vi "MeasureSave.vi"(7 "MinutesToWait":u32, 8 "Stop":bool, 9 "Number of Spectra":u16=1, 11 "Handle":u32) -> (1 "phase":dbl[](array[numeric]), 2 "mag":dbl[](array[numeric]), 3 "Freq":dbl[](array[numeric]), 4 "Current Incoming row":u16, 6 "SpecCount":u16)   [LabVIEW 2012]
uses:
  <vilib>/Utility/file.llb/Write To Spreadsheet File (DBL).vi
  Sciospec ISX3 Impedance Analyzer.lvlib
panel:
  out "ACK for Start CMD":u8[](array[numeric])
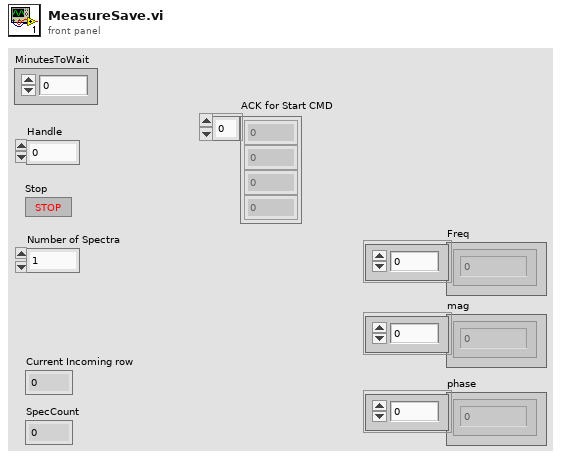
[diagram p1: front panel]
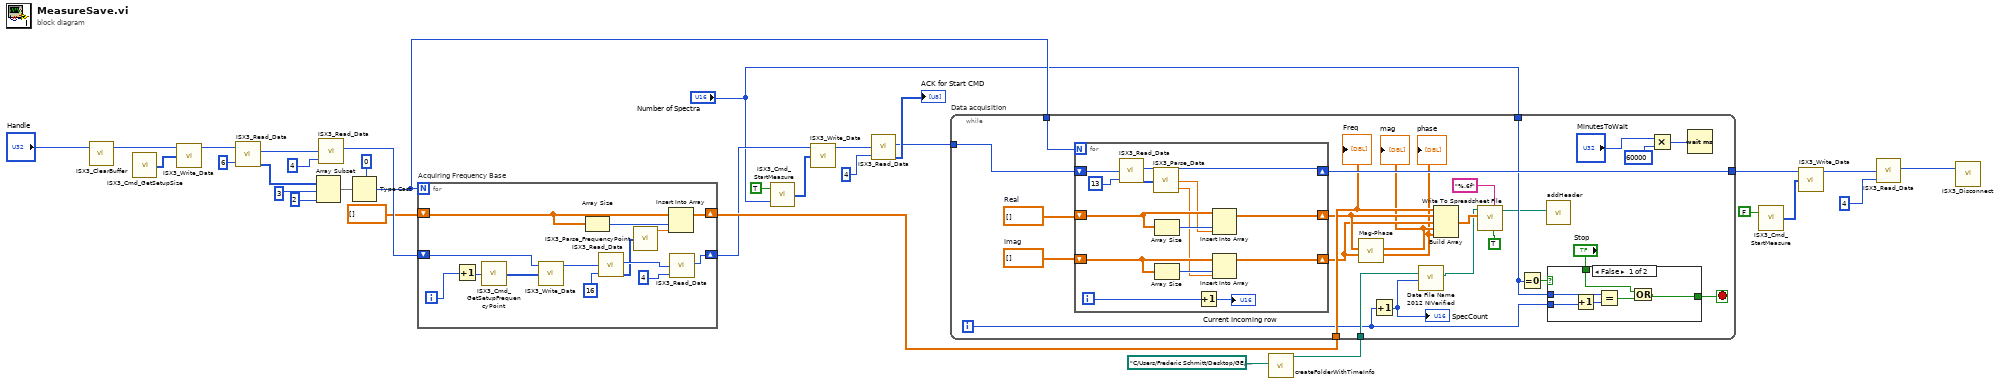
[diagram p0: block diagram]
diagram:
  n1 = call "ISX3_ClearBuffer.vi"("Handle"="Handle") -> ("Handle"=w4:u32)  [unwired: 1 in, 1 out]
  n2 = call "ISX3_Cmd_GetSetupSize.vi"() -> ("get Setup Size Cmd"=w15:u8[])  [unwired: 1 in]
  n3 = call "ISX3_Write_Data.vi"("Data to Write"=w15, "FT_Handle"=w4) -> ("FT_Handle"=w16:u32)  [unwired: 2 in, 1 out]
  n4 = call "ISX3_Read_Data.vi"("FT_Handle"=w16, "Bytes To Read"=6) -> ("Handle"=w27:u32, "Read Data"=w25:u8[])  [unwired: 2 in, 1 out]
  n5 = Array Subset(array=w25, index=3, length=2) -> (w26:u8[])
  n6 = call "ISX3_Read_Data.vi"("FT_Handle"=w27, "Bytes To Read"=4) -> ("Handle"=w21:u32)  [unwired: 2 in, 2 out]
  n7 = Type Cast(type=u16 0, x=w26) -> (*(type *) &x=w18:u16)
  n8 = for "Acquiring Frequency Base" {
    N: w18 -> [_]
    shift-right: [w42] -> w20
    shift-left: dbl[] [] -> [w43]
    shift-right: [w39] -> w14
    shift-left: w21 -> [w37]
    i -> [w46]
    n9 = Increment(x=w46) -> (x+1=w38:i32)
    n10 = call "ISX3_Cmd_GetSetupFrequencyPoint.vi"("Row"=w38) -> ("get Setup Frequency Point Cmd"=w36:u8[])
    n11 = call "ISX3_Write_Data.vi"("Data to Write"=w36, "FT_Handle"=w37) -> ("FT_Handle"=w35:u32)  [unwired: 2 in, 1 out]
    n12 = Array Size(array=w43) -> (size(s)=w44:i32)
    n13 = call "ISX3_Read_Data.vi"("FT_Handle"=w35, "Bytes To Read"=16) -> ("Handle"=w41:u32, "Read Data"=w34:u8[])  [unwired: 2 in, 1 out]
    n14 = call "ISX3_Parse_FrequencyPoint.vi"("Array"=w34) -> ("Frequency [Hz]"=w33:sgl)  [unwired: 2 out]
    n15 = Insert Into Array(array=w43, index=w44, new element=w33) -> (w42:dbl[])
    n16 = call "ISX3_Read_Data.vi"("FT_Handle"=w41, "Bytes To Read"=4) -> ("Handle"=w39:u32)  [unwired: 2 in, 2 out]
  }
  n17 = call "ISX3_Cmd_StartMeasure.vi"("Number of Spectra"="Number of Spectra", "Start/Stop"=TRUE) -> ("Start/Stop measurement cmd"=w10:u8[])
  n18 = call "ISX3_Write_Data.vi"("Data to Write"=w10, "FT_Handle"=w14) -> ("FT_Handle"=w13:u32)  [unwired: 2 in, 1 out]
  n19 = call "ISX3_Read_Data.vi"("FT_Handle"=w13, "Bytes To Read"=4) -> ("Handle"=w30:u32, "Read Data"=→"ACK for Start CMD":u8[])  [unwired: 2 in, 1 out]
  n20 = call "createFolderWithTimeInfo.vi"("Folder to save file to"=path "C:/Users/Frederic Schmitt/Desktop/GE/Sciospec Bioimpedance - Sinan/Sciospec ISX3v2/Data from LabVIEW") -> ("created path"=w3:path)  [unwired: 10 in]
  n21 = while "Data acquisition" {
    tunnel: w30 -> [w71]
    tunnel: [w68] -> w7
    tunnel: w20 -> [w62]
    tunnel: "Number of Spectra" -> [w66]
    tunnel: w18 -> [w63]
    tunnel: w3 -> [w58]
    i -> [w51]
    stop <- w65 stop-if-true
    w69 = dbl[] []  # Imag
    w70 = dbl[] []  # Real
    n22 = for {
      N: w63 -> [_]
      shift-right: [w91] -> w68
      shift-left: w71 -> [w92]
      shift-right: [w86] -> w56
      shift-left: w70 -> [w84]
      shift-right: [w88] -> w55
      shift-left: w69 -> [w89]
      i -> [w83]
      n23 = call "ISX3_Read_Data.vi"("FT_Handle"=w92, "Bytes To Read"=13) -> ("Handle"=w91:u32, "Read Data"=w79:u8[])  [unwired: 2 in, 1 out]
      n24 = call "ISX3_Parse_Data.vi"("Array"=w79) -> ("Real"=w81:sgl, "Imag"=w80:sgl)  [unwired: 1 out]
      n25 = Array Size(array=w84) -> (size(s)=w87:i32)
      n26 = Array Size(array=w89) -> (size(s)=w90:i32)
      n27 = Increment(x=w83) -> (x+1=→"Current Incoming row":i32)
      n28 = Insert Into Array(array=w84, index=w87, new element=w81) -> (w86:dbl[])
      n29 = Insert Into Array(array=w89, index=w90, new element=w80) -> (w88:dbl[])
    }
    n30 = call "Mag-Phase.vi"("Imag"=w55, "Re"=w56) -> ("phase"=w53:dbl[], "mag"=w54:dbl[])  [unwired: 7 in]
    "mag" <- w54
    "phase" <- w53
    n31 = Increment(x=w51) -> (x+1=w50:i32)
    "SpecCount" <- w50
    n32 = call "Date File Name 2012 NIVerified.vi"("Data Count"=w50, "Folder to save file to"=w58) -> ("New file path"=w59:path)  [unwired: 9 in]
    n33 = Build Array(w62, w56, w55, w54, w53) -> (w61:dbl[][])
    n34 = call-poly <vilib>:"Write To Spreadsheet File.vi"("transpose? (no:F)"=TRUE, "format (%.3f)"="%.6f", "2D data"=w61, "file path (dialog if empty)"=w59) -> ("new file path (Not A Path if cancelled)"=w57:path)  [unwired: 4 in]
    n35 = Equal To 0?(x=w66) -> (x = 0?=w67:bool)
    n36 = call "addHeader.vi"("file path (dialog if empty)"=w57) -> ()  [unwired: 11 in]
    n37 = case shown="False" w67 {
      tunnel: w66 -> [w77 _]
      tunnel: w51 -> [w76 _]
      tunnel: [w74 w78] -> w65
      tunnel: "Stop" -> [w73 w78]
      frame False {
        n38 = Increment(x=w76) -> (x+1=w75:i32)
        n39 = Equal?(x=w77, y=w75) -> (x = y?=w72:bool)
        n40 = Or(x=w73, y=w72) -> (x .or. y?=w74:bool)
      }
      frame True {
      }
    }
    n41 = Multiply(x="MinutesToWait", y=u32 60000) -> (x*y=w48:u32)
    n42 = Wait (ms)(milliseconds to wait=w48) -> ()  [unwired: 1 out]
    "Freq" <- w62
  }
  n43 = call "ISX3_Cmd_StartMeasure.vi"("Start/Stop"=FALSE) -> ("Start/Stop measurement cmd"=w8:u8[])  [unwired: 1 in]
  n44 = call "ISX3_Write_Data.vi"("Data to Write"=w8, "FT_Handle"=w7) -> ("FT_Handle"=w6:u32)  [unwired: 2 in, 1 out]
  n45 = call "ISX3_Read_Data.vi"("FT_Handle"=w6, "Bytes To Read"=4) -> ("Handle"=w5:u32)  [unwired: 2 in, 2 out]
  n46 = call "ISX3_Disconnect.vi"("FT_Handle"=w5) -> ()  [unwired: 2 in]
